vi "Pomodoro.vi"() -> ()   [LabVIEW 2010]
panel:
  in  "Sound File":path
  in  "Play Sound File":bool
  in  "Period Type":enum16{"Pomodoro", "Short Break", "Long Break"}(ring)
  in  "Start":bool
  in  "Timer (HH:MM:SS)":string="00:00:10"
  in  "Exit":bool
  in  "Stop":bool
  out "Running?":bool
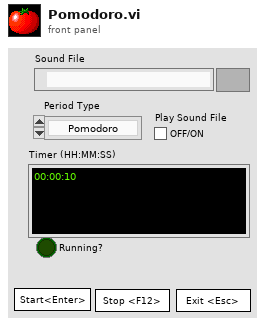
[diagram p1: front panel]
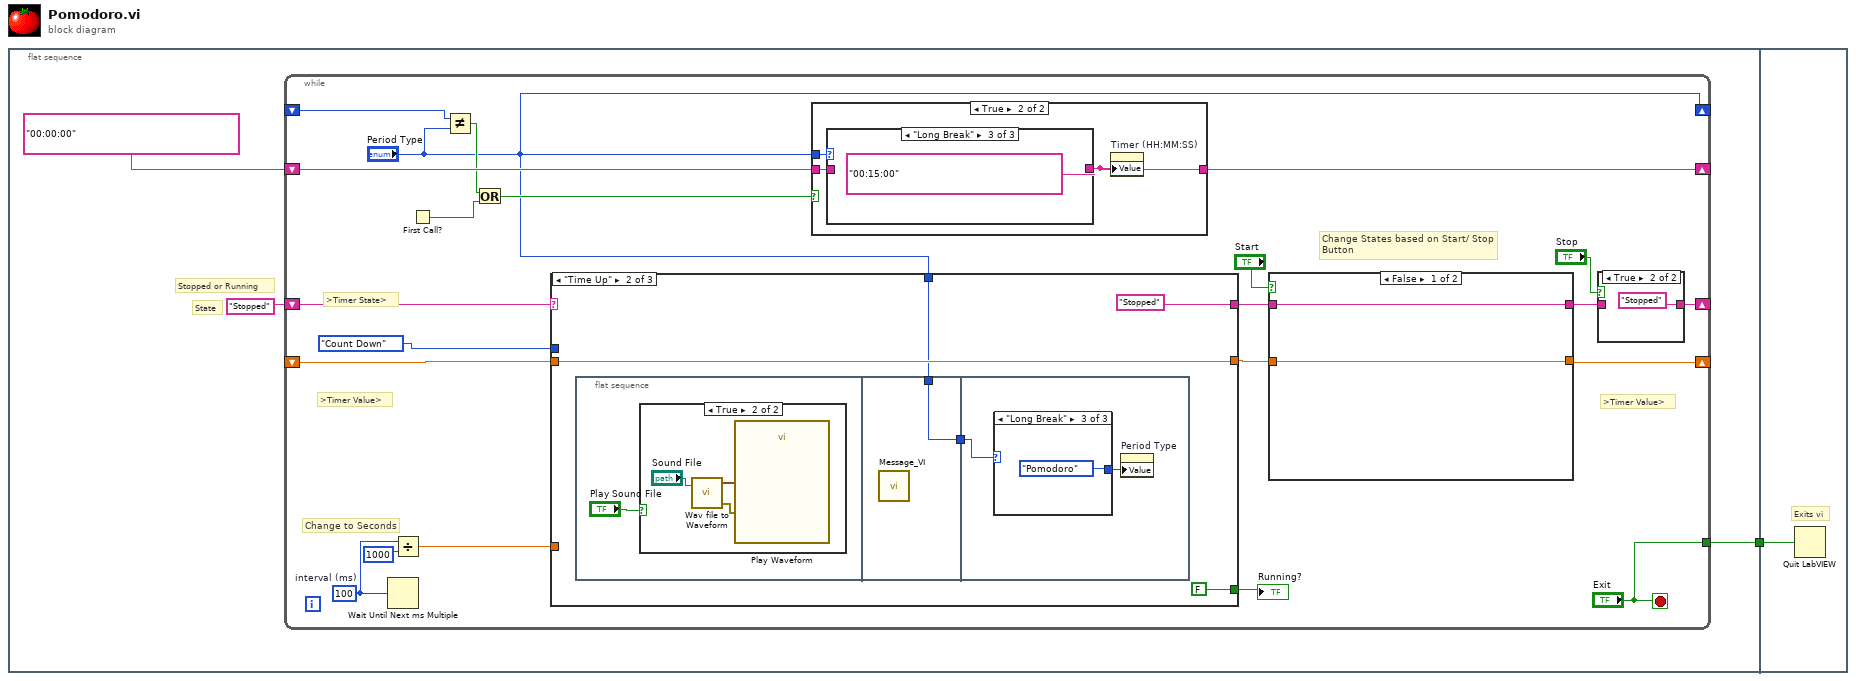
[diagram p0: block diagram]
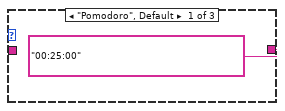
[diagram p3: hidden frame]
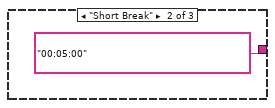
[diagram p4: hidden frame]
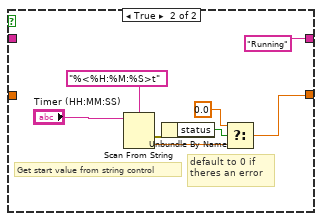
[diagram p6: hidden frame]
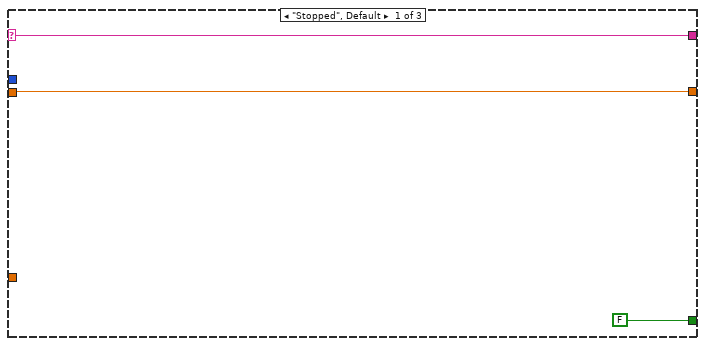
[diagram p7: hidden frame]
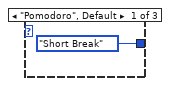
[diagram p9: hidden frame]
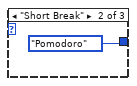
[diagram p10: hidden frame]
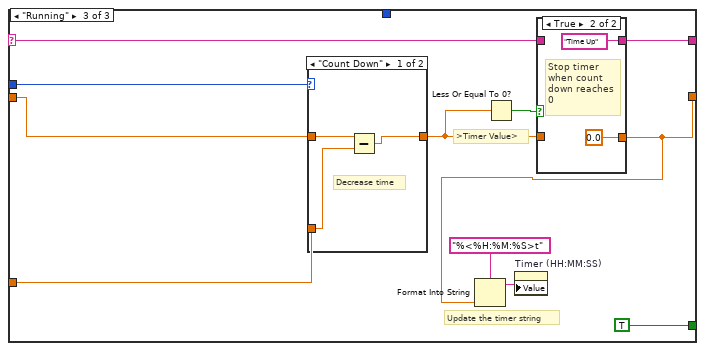
[diagram p11: hidden frame]
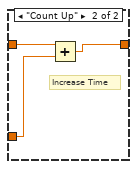
[diagram p13: hidden frame]
diagram:
  n1 = flat-sequence {
    tunnel: [w2] -> w1
    tunnel: w1 -> [w85]
    frame #0 {
      # "Stopped or Running"
      # "State"
      n2 = while {
        shift-right: [w22] -> _
        shift-left: "Stopped" -> [w26]
        shift-right: [w21] -> _
        shift-left: _ -> [w20]
        shift-right: [w12] -> _
        shift-left: "00:00:00" ("Text.Text") -> [w11]
        shift-right: ["Period Type"] -> _
        shift-left: _ -> [w10]
        tunnel: ["Exit"] -> w2
        stop <- "Exit" stop-if-true
        w18 = u32 100  # interval (ms)
        # ">Timer Value>"
        # ">Timer Value>"
        # ">Timer State>"
        # "Change to Seconds"
        # "Change States based on Start/ Stop\nButton"
        n3 = Wait Until Next ms Multiple(millisecond multiple=w18) -> ()  [unwired: 1 out]
        n4 = Divide(x=w18, y=u32 1000) -> (x/y=w16:dbl)
        n5 = First Call?() -> (First Call?: T/F=w9:bool)
        n6 = Not Equal?(x=w10, y="Period Type") -> (x != y?=w8:bool)
        n7 = Or(x=w8, y=w9) -> (x .or. y?=w7:bool)
        n8 = case shown="\"Time Up\"" w26 {
          selector: w26 -> [w47 _ w68]
          tunnel: w20 -> [w46 w52 w73]
          tunnel: enum32{"Count Up", "Count Down"}."Count Down" ("Counter Mode") -> [_ _ w74]
          tunnel: [w46 w52 w64] -> w19
          tunnel: w16 -> [_ _ w72]
          tunnel: [FALSE ("Running?") FALSE ("Running?") TRUE ("Running?")] -> w15
          tunnel: [w47 "Stopped" w65] -> w14
          tunnel: "Period Type" -> [_ w49 _]
          frame "Stopped", Default {
          }
          frame "Time Up" {
            n9 = flat-sequence {
              tunnel: [w58] -> w50
              tunnel: w49 -> [w58]
              tunnel: w50 -> [w60]
              frame #0 {
                n10 = case shown="True" "Play Sound File" {
                  frame False {
                  }
                  frame True {
                    n11 = call "Wav file to Waveform.vi"("Path"="Sound File") -> ("error out"=w57:errorcluster, "Output Waveform"=w56:waveform(dbl))  [unwired: 1 in, 1 out]
                    n12 = call "Play Waveform"("Data"=w56, "error in"=w57) -> ()  [unwired: 17 in, 1 out]
                  }
                }
              }
              frame #1 {
                n13 = call "Message_VI.vi"() -> ()  [unwired: 12 in]
              }
              frame #2 {
                n14 = case shown="\"Long Break\"" w60 {
                  tunnel: [enum16{"Pomodoro", "Short Break", "Long Break"}."Short Break" ("Period Type") enum16{"Pomodoro", "Short Break", "Long Break"}."Pomodoro" ("Period Type") enum16{"Pomodoro", "Short Break", "Long Break"}."Pomodoro" ("Period Type")] -> w59
                  frame "Pomodoro", Default {
                  }
                  frame "Short Break" {
                  }
                  frame "Long Break" {
                  }
                }
                n15 = property on="Period Type" class="Enum (strict)"("Value"=w59) -> ()  [unwired: 2 in, 2 out]
              }
            }
          }
          frame "Running" {
            # ">Timer Value>"
            # "Update the timer string"
            n16 = case shown="\"Count Down\"" w74 {
              tunnel: w73 -> [w81 w84]
              tunnel: [w79 w83] -> w67
              tunnel: w72 -> [w80 w82]
              frame "Count Down" {
                # "Decrease time"
                n17 = Subtract(x=w81, y=w80) -> (x-y=w79:dbl)
              }
              frame "Count Up" {
                # "Increase Time"
                n18 = Add(x=w84, y=w82) -> (x+y=w83:dbl)
              }
            }
            n19 = Less Or Equal To 0?(x=w67) -> (x <= 0?=w66:bool)
            n20 = case shown="True" w66 {
              tunnel: w67 -> [w75 _]
              tunnel: [w75 0.0 ("t")] -> w64
              tunnel: w68 -> [w76 _]
              tunnel: [w76 "Time Up"] -> w65
              frame False {
              }
              frame True {
                # "Stop timer when count down reaches 0"
              }
            }
            n21 = Format Into String(format string="%<%H:%M:%S>t", w64) -> (resulting string=w71:string)  [unwired: 2 in, 1 out]
            n22 = property on="Timer (HH:MM:SS)" class="Str"("Value"=w71) -> ()  [unwired: 2 in, 2 out]
          }
        }
        "Running?" <- w15
        n23 = case shown="True" w7 {
          tunnel: [w27 w30] -> w12
          tunnel: w11 -> [w27 w29]
          tunnel: "Period Type" -> [_ w28]
          frame False {
          }
          frame True {
            n24 = case shown="\"Long Break\"" w28 {
              tunnel: ["00:25:00" ("Text.Text") "00:05:00" ("Text.Text") "00:15:00" ("Text.Text")] -> w30
              tunnel: w29 -> [_ _ _]
              frame "Pomodoro", Default {
              }
              frame "Short Break" {
              }
              frame "Long Break" {
              }
            }
            n25 = property on="Timer (HH:MM:SS)" class="Str"("Value"=w30) -> ()  [unwired: 2 in, 2 out]
          }
        }
        n26 = case shown="False" "Start" {
          tunnel: [w37 "Running"] -> w23
          tunnel: w14 -> [w37 _]
          tunnel: [w36 w39] -> w21
          tunnel: w19 -> [w36 _]
          frame False {
          }
          frame True {
            # "default to 0 if theres an error"
            # "Get start value from string control"
            n27 = Scan From String(format string="%<%H:%M:%S>t", input string="Timer (HH:MM:SS)") -> (error out=w42:errorcluster, output 1=w40:dbl)  [unwired: 3 in, 2 out]
            n28 = Unbundle By Name(w42) -> ("status"=w38:bool)
            n29 = Select(t=0.0, s=w38, f=w40) -> (s? t:f=w39:dbl)
          }
        }
        n30 = case shown="True" "Stop" {
          tunnel: [w34 "Stopped"] -> w22
          tunnel: w23 -> [w34 _]
          frame False {
          }
          frame True {
          }
        }
      }
    }
    frame #1 {
      # "Exits vi"
      n31 = Quit LabVIEW(quit? (T)=w85) -> ()
    }
  }
